vi "AiTo64Bit.vi"(1 "AI 3":i16, 2 "AI 2":i16, 3 "AI 1":i16, 4 "AI 0":i16) -> (0 "AI 64bit":i64)   [LabVIEW 2014]
doc: "Converts four I16 int to one I64.\nUsed to bundle 4 analog input samples to one 64 bit input for the DRAM."
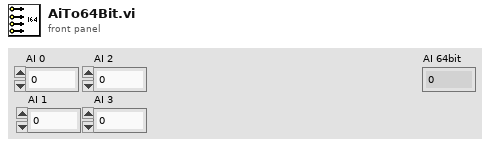
[diagram p1: front panel]
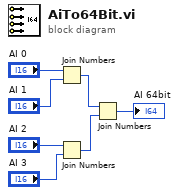
[diagram p0: block diagram]
diagram:
  n1 = Join Numbers(hi="AI 0", lo="AI 1") -> ((hi.lo)=w7:u32)
  n2 = Join Numbers(hi="AI 2", lo="AI 3") -> ((hi.lo)=w6:u32)
  n3 = Join Numbers(hi=w7, lo=w6) -> ((hi.lo)=→"AI 64bit":u64)
